vi "Set AccessType.vi"(8 "error in":errorcluster, 10 "Value":refnum<class "Value.lvclass">, 11 "Object Type in":refnum<class "Object Type Base.lvclass">) -> (0 "error out":errorcluster, 3 "Object Type out":refnum<class "Object Type Base.lvclass">)   [LabVIEW 2024, in "Electronic Datasheet.lvlib" / "Object Type Base.lvclass"]
uses:
  Object Type Base.lvclass
  Value/Value.lvclass
  Object Type Base.lvclass/Object Type Base.ctl
  Electronic Datasheet.lvlib
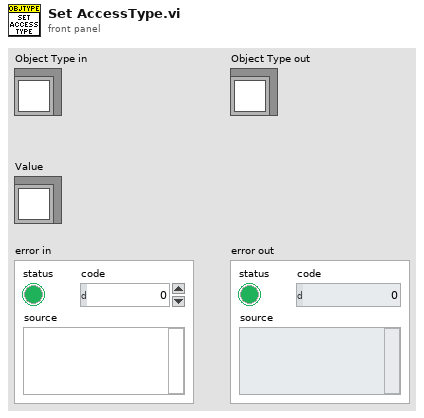
[diagram p1: front panel]
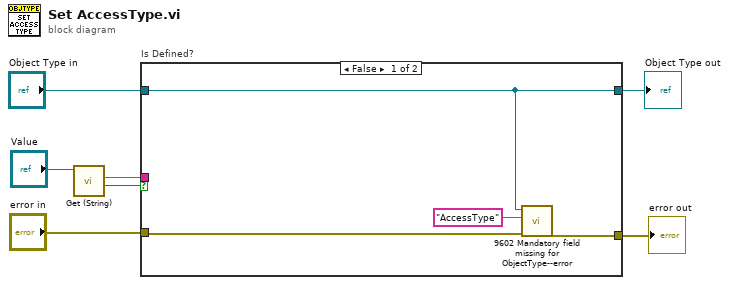
[diagram p0: block diagram]
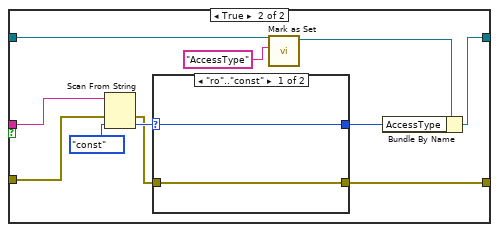
[diagram p2: hidden frame]
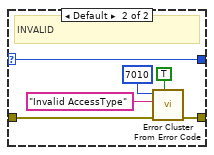
[diagram p3: hidden frame]
diagram:
  n1 = call "Get (String).vi"("Value in"="Value") -> ("Defined?"=w4:bool, "Value"=w3:string)  [unwired: 8 in, 1 out]
  n2 = case "Is Defined?" shown="False" w4 {
    tunnel: [w9 w22] -> w7
    tunnel: "Object Type in" -> [w9 w21]
    tunnel: w3 -> [_ w15]
    tunnel: [w10 w17] -> w2
    tunnel: "error in" -> [w8 w13]
    frame False {
      n3 = call "9602 Mandatory field missing for ObjectType--error.vi"("error in"=w8, "Field Name"="AccessType" ("error message (\"\")"), "Object Type Base"=w9) -> ("error out"=w10:errorcluster)  [unwired: 8 in]
    }
    frame True {
      n4 = Scan From String(input string=w15, error in=w13, default 1=enum16{"ro", "wo", "rw", "rwr", "rww", "const"}."const" ("AccessType")) -> (error out=w12:errorcluster, output 1=w14:enum16{"ro", "wo", "rw", "rwr", "rww", "const"})  [unwired: 2 in, 2 out]
      n5 = case shown="\"ro\"..\"const\"" w14 {
        selector: w14 -> [w24 w29]
        tunnel: [w23 w30] -> w17
        tunnel: [w24 w29] -> w18
        tunnel: w12 -> [w23 w25]
        frame "ro".."const" {
        }
        frame Default {
          # "INVALID"
          n6 = call <vilib>:"Error Cluster From Error Code.vi"("show call chain? (False)"=TRUE, "error in (no error)"=w25, "error message (\"\")"="Invalid AccessType" ("error message (\"\")"), "error code (0)"=7010) -> ("error out"=w30:errorcluster)  [unwired: 5 in]
        }
      }
      n7 = call "Mark as Set.vi"("Field name"="AccessType", "Object Type in"=w21) -> ("Object Type out"=w20:refnum<class "Object Type Base.lvclass">)  [unwired: 9 in]
      n8 = Bundle By Name(cluster=w20, "AccessType"=w18) -> (w22:refnum<class "Object Type Base.lvclass">)
    }
  }
  "Object Type out" <- w7
  "error out" <- w2
